vi "MeasurementServer_SetResponse_Invoke.vi"(0 "gRPCid":T1, 2 "status":i32, 3 "error in (no error)":errorcluster) -> (10 "error out":errorcluster)   [LabVIEW 2019, in "labview-grpc-measurement-server.lvlib"]
uses:
  labview-grpc-measurement-server.lvlib
  MeasurementServer_gRPCid.ctl
  MeasurementServer_InvokeResponse.ctl
  build/Release/labview_measurement_server.dll
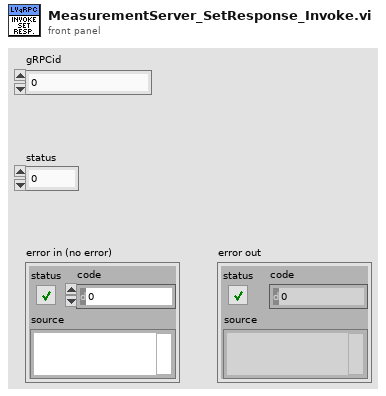
[diagram p1: front panel]
types:
  T1 = typedef "labview-grpc-measurement-server.lvlib/MeasurementServer_gRPCid.ctl" = u64
  T2 = typedef "labview-grpc-measurement-server.lvlib/MeasurementServer_InvokeResponse.ctl" = cluster{"status":i32}
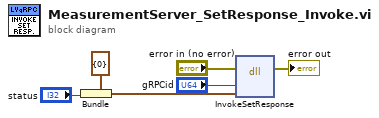
[diagram p0: block diagram]
diagram:
  n1 = Bundle(cluster=T2 {"status"=0} ("InvokeResponse"), "status"="status") -> (w3:T2)
  n2 = dll-call lib="C:/Users/chericks/Desktop/LabVIEW-grpc-measurement-server/build/Release/labview_measurement_server.dll" fn="InvokeSetResponse"(error in="error in (no error)", "id"="gRPCid", "data"=w3) -> (error out=→"error out":errorcluster)  [unwired: 5 in, 1 out]
